vi "Sequence - Action Test.vi"(8 "error in (no error)":errorcluster, 11 "Test":string) -> (0 "error out":errorcluster)   [LabVIEW 2020]
uses:
  Library - Test Executive.llb/Test Executive - Globals.vi
  Library - Test Executive.llb/Test Executive.lvlib
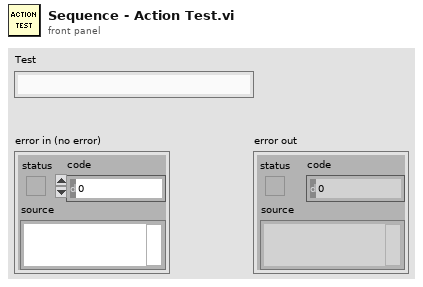
[diagram p1: front panel]
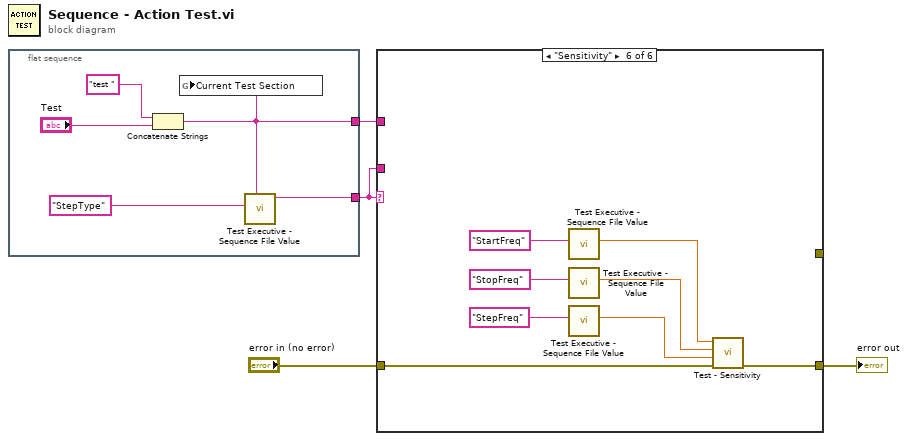
[diagram p0: block diagram]
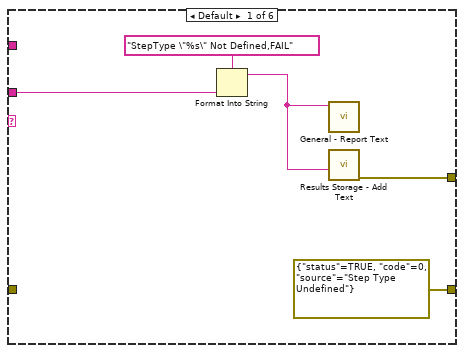
[diagram p2: hidden frame]
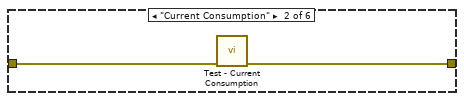
[diagram p3: hidden frame]
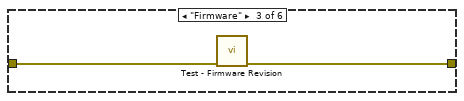
[diagram p4: hidden frame]
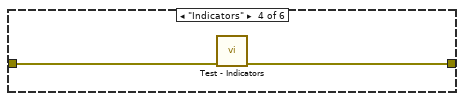
[diagram p5: hidden frame]
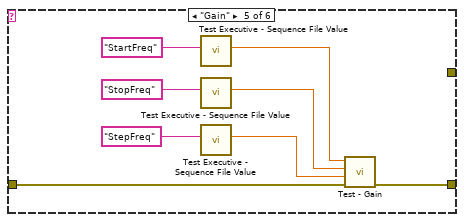
[diagram p6: hidden frame]
diagram:
  n1 = flat-sequence {
    tunnel: [w6] -> w1
    tunnel: [w5] -> w2
    frame #0 {
      n2 = Concatenate Strings("test ", "Test") -> (w5:string)
      n3 = global write "Test Executive - Globals.vi" "Current Test Section"(w5) -> ()
      n4 = call "Test Executive - Sequence File Value.vi"("Section (Current Test)"=w5, "Key"="StepType") -> ("String"=w6:string)  [unwired: 6 in, 3 out]
    }
  }
  n5 = case shown="\"Sensitivity\"" w1 {
    tunnel: "error in (no error)" -> [_ w16 w18 w20 w28 w32]
    tunnel: [errorcluster {"status"=TRUE, "code"=0, "source"="Step Type Undefined"} ("error out") w15 w17 w19 w27 w36] -> w3
    tunnel: [w11 _ _ _ _ _] -> _
    tunnel: w2 -> [_ _ _ _ _ _]
    tunnel: w1 -> [w10 _ _ _ _ _]
    frame Default {
      n6 = Format Into String(format string="StepType \"%s\" Not Defined,FAIL" ("Text In"), w10) -> (resulting string=w12:string)  [unwired: 2 in, 1 out]
      n7 = call "General - Report Text.vi"("Text In"=w12) -> ()  [unwired: 8 in, 3 out]
      n8 = call "Results Storage - Add Text.vi"("Text"=w12) -> ("error out"=w11:errorcluster)  [unwired: 10 in]
    }
    frame "Current Consumption" {
      n9 = call "Test - Current Consumption.vi"("error in (no error)"=w16) -> ("error out"=w15:errorcluster)  [unwired: 10 in]
    }
    frame "Firmware" {
      n10 = call "Test - Firmware Revision.vi"("error in (no error)"=w18) -> ("error out"=w17:errorcluster)  [unwired: 10 in]
    }
    frame "Indicators" {
      n11 = call "Test - Indicators.vi"("error in (no error)"=w20) -> ("error out"=w19:errorcluster)  [unwired: 10 in]
    }
    frame "Gain" {
      n12 = call "Test Executive - Sequence File Value.vi"("Key"="StartFreq") -> ("Numeric Value"=w23:dbl)  [unwired: 7 in, 3 out]
      n13 = call "Test Executive - Sequence File Value.vi"("Key"="StopFreq") -> ("Numeric Value"=w22:dbl)  [unwired: 7 in, 3 out]
      n14 = call "Test Executive - Sequence File Value.vi"("Key"="StepFreq") -> ("Numeric Value"=w21:dbl)  [unwired: 7 in, 3 out]
      n15 = call "Test - Gain.vi"("error in (no error)"=w28, "Step Frequency"=w21, "Stop Frequency"=w22, "Start Frequency"=w23) -> ("error out"=w27:errorcluster)  [unwired: 7 in]
    }
    frame "Sensitivity" {
      n16 = call "Test Executive - Sequence File Value.vi"("Key"="StartFreq") -> ("Numeric Value"=w31:dbl)  [unwired: 7 in, 3 out]
      n17 = call "Test Executive - Sequence File Value.vi"("Key"="StopFreq") -> ("Numeric Value"=w30:dbl)  [unwired: 7 in, 3 out]
      n18 = call "Test Executive - Sequence File Value.vi"("Key"="StepFreq") -> ("Numeric Value"=w29:dbl)  [unwired: 7 in, 3 out]
      n19 = call "Test - Sensitivity.vi"("error in (no error)"=w32, "Step Frequency"=w29, "Stop Frequency"=w30, "Start Frequency"=w31) -> ("error out"=w36:errorcluster)  [unwired: 7 in]
    }
  }
  "error out" <- w3
